vi "Teleop.vi"(10 "Match Info":T4={"Autonomous Elapsed Seconds"=0.0, "TeleOp Elapsed Seconds"=0.0, "Disabled Elapsed Seconds"=0.0, "Visited Autonomous"=FALSE, "Visited TeleOp"=FALSE, "Visited Disabled"=FALSE, "Autonomous Settings"={"Autonomous Style"=enum."Independent", "VI Refnum"=refnum}}, 11 "Call Context":T5) -> ()   [LabVIEW 2020]
doc: "This VI is called for each TeleOp packet received from the DS where the robot is not disabled. It is often used to read from the joysticks and update I/O or to update setpoints for timed control loops. It should complete and return within 20 milliseconds or it may miss DS packets."
uses:
  <vilib>/Rock Robotics/WPI/DriverStation/WPI_DriverStationDerivedRobotMode.ctl
  <vilib>/Rock Robotics/WPI/DriverStation/WPI_DriverStationMatch Info.ctl
  <vilib>/Rock Robotics/WPI/ThirdParty/REV Robotics/REVLib/Typedef/Color Sensor V3 Resolution.ctl
  <vilib>/Rock Robotics/WPI/ThirdParty/REV Robotics/REVLib/Typedef/Color Sensor V3 MeasurementRate.ctl
  <vilib>/Rock Robotics/WPI/ThirdParty/REV Robotics/REVLib/Typedef/Color Sensor V3 GainFactor.ctl
  <vilib>/Rock Robotics/WPI/ThirdParty/Phoenix-LabVIEW/Motor Controller/Controls/CTRE_Phoenix_MotorControl_ControlMode.ctl
  <vilib>/Rock Robotics/Network Tables/NT Read Boolean.vi
  <vilib>/Rock Robotics/Network Tables/NT Read Number.vi
  <vilib>/Rock Robotics/WPI/Utilities/WPI_GetSetVariantRefNum.vi
  GitHub/2022-Rapid-React-Code/TitanLib/Lib/TitanLib.lvlib
  <vilib>/Rock Robotics/WPI/ThirdParty/Phoenix-LabVIEW/CANCoder/Get/CTRE_Phoenix_CANcoder_GetSensorData.vi
panel:
  in  "Azimuth Limit":dbl(slide) scale=0.0..1.0
  in  "Drive Limit":dbl(slide) scale=0.0..1.0
  out "IR Detected":bool
  in  "Set":bool
  in  "GainFactor":T1
  in  "ColorSensorMeasurementRate":T2
  in  "ColorSensorResolution":T3
  in  "Red Calibration":cluster{"R":dbl, "G":dbl, "B":dbl}
  in  "Blue Calibration":cluster{"R":dbl, "G":dbl, "B":dbl}
  in  "Yellow Calibration":cluster{"R":dbl, "G":dbl, "B":dbl}
  in  "Green Calibration":cluster{"R":dbl, "G":dbl, "B":dbl}
  out "Proximity Chart":u16(graph)
  out "Confidence":dbl
  out "Matched Color Name":string
  out "error out":errorcluster
  out "Color":u32(colorbox)
  out "Measured Color":cluster{"R":dbl, "G":dbl, "B":dbl}
  out "Sample Slider 0":dbl(slide) scale=0.0..5.0
  out "Sample Boolean 1":bool
  out "Sample Boolean 0":bool
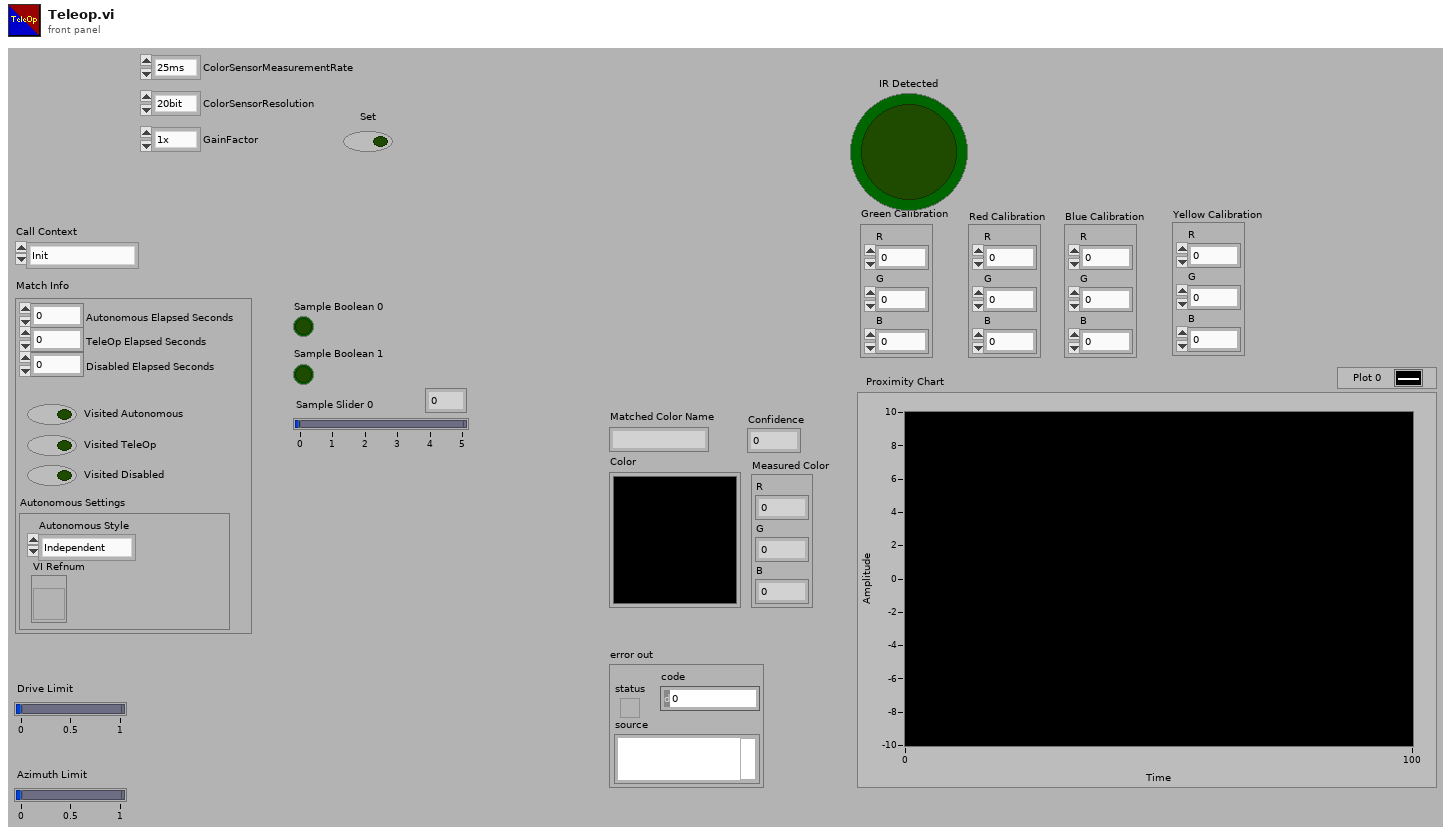
[diagram p1: front panel]
types:
  T1 = typedef "Color Sensor V3 GainFactor.ctl" = enum16{"1x", "3x", "6x", "9x", "18x"}
  T2 = typedef "Color Sensor V3 MeasurementRate.ctl" = enum16{"25ms", "50ms", "100ms", "200ms", "500ms", "1000ms", "2000ms"}
  T3 = typedef "Color Sensor V3 Resolution.ctl" = enum16{"20bit", "19bit", "18bit", "17bit", "16bit", "13bit"}
  T4 = typedef "WPI_DriverStationMatch Info.ctl" = cluster{"Autonomous Elapsed Seconds":dbl, "TeleOp Elapsed Seconds":dbl, "Disabled Elapsed Seconds":dbl, "Visited Autonomous":bool, "Visited TeleOp":bool, "Visited Disabled":bool, "Autonomous Settings":cluster{"Autonomous Style":enum16{"Iterative", "Independent"}, "VI Refnum":refnum<vi>}}
  T5 = typedef "WPI_DriverStationDerivedRobotMode.ctl" = enum16{"Init", "Execute", "Stop"}
  T6 = typedef "CTRE_Phoenix_MotorControl_ControlMode.ctl" = u16
  T7 = typedef "Color Sensor V3 DevRef.ctl" = cluster{"I2CDevRef":T8}
  T8 = typedef "WPI_I2CDevRef.ctl" = cluster{"DevStatus":errorcluster, "Device Address":u8, "Handle":i32, "I2C Bus":T9}
  T9 = typedef "i2c_bus.ctl" = enum16{"I2C On-Board", "I2C MXP", "Invalid"}
  T10 = typedef "WPI_DigitalInputDevRef.ctl" = cluster{"DevStatus":errorcluster, "DIO Channel":T11}
  T11 = typedef "FPGA_DIOChannel.ctl" = enum8{"DIO 0", "DIO 1", "DIO 2", "DIO 3", "DIO 4", "DIO 5", "DIO 6", "DIO 7", "DIO 8", "DIO 9", "DIO MXP 0", "DIO MXP 1", "DIO MXP 2", "DIO MXP 3", "DIO MXP 4", "DIO MXP 5", "DIO MXP 6", "DIO MXP 7", "DIO MXP 8", "DIO MXP 9", "DIO MXP 10", "DIO MXP 11", "DIO MXP 12", "DIO MXP 13", "DIO MXP 14", "DIO MXP 15", "SPI Port CS1", "SPI Port CS2", "SPI Port CS3", "SPI Port MISO", "SPI Port MOSI", "Invalid"}
  T12 = typedef "WPI_JoystickDevRef.ctl" = cluster{"Device":T13}
  T13 = typedef "WPI_JoystickDeviceEnum.ctl" = enum16{"USB 0", "USB 1", "USB 2", "USB 3", "USB 4", "USB 5"}
  T14 = typedef "CTRE_Phoenix_CANcoder_DeviceRef.ctl" = cluster{"DeviceStatus":errorcluster, "Device Number":u8, "Handle":u64, "UsageFrame":u32, "Library Path":path}
  T15 = typedef "WPI_MotorControlDeviceRef.ctl" = cluster{"DeviceStatus":errorcluster, "Type":T16, "PWM":cluster{"PWM Channel":T17, "DeadBand":T18}, "CAN":cluster{"Device Number":u8, "SetOutput VI Ref":variant, "GetOutput VI Ref":variant, "Enable VI Ref":variant, "Disable VI Ref":variant, "Data":variant}, "Invert":bool, "DIO PWM":cluster{"PWM \"Enable\" Channel":T17, "DIOChannel":T11, "PWM Rate":dbl}}
  T16 = typedef "WPI_MotorControlType.ctl" = enum16{"PWM", "CAN", "DIO PWM"}
  T17 = typedef "FPGA_DIOPWMChannel.ctl" = enum8{"PWM 0", "PWM 1", "PWM 2", "PWM 3", "PWM 4", "PWM 5", "PWM 6", "PWM 7", "PWM 8", "PWM 9", "PWM MXP 0", "PWM MXP 1", "PWM MXP 2", "PWM MXP 3", "PWM MXP 4", "PWM MXP 5", "PWM MXP 6", "PWM MXP 7", "PWM MXP 8", "PWM MXP 9", "Invalid"}
  T18 = typedef "WPI_PWMDeadband.ctl" = cluster{"Name":string, "maxPositivePwm":i32, "minPositivePwm":i32, "centerPwm":i32, "maxNegativePwm":i32, "minNegativePwm":i32, "angularRange":u16}
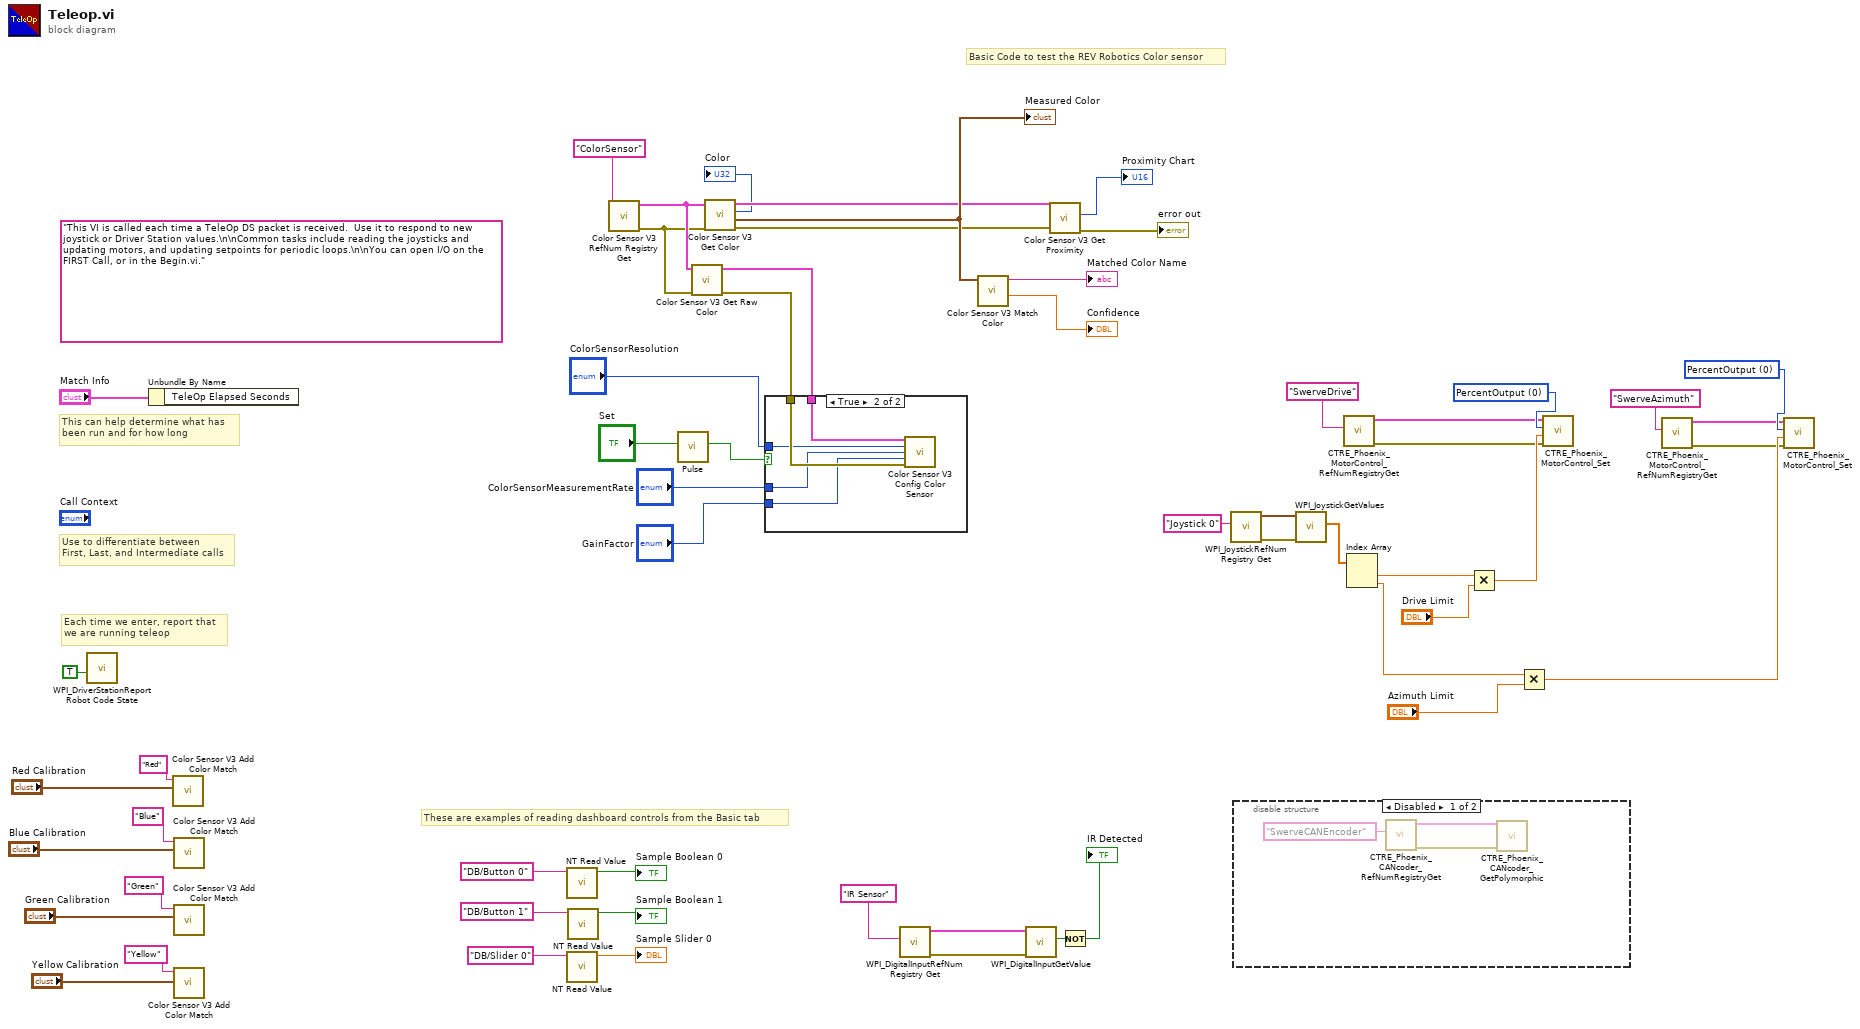
[diagram p0: block diagram]
diagram:
  w18 = T6 0 items=["PercentOutput"=0, "Position"=1, "Velocity"=2, "Current"=3, "Follower"=5, "MotionProfile"=6, "MotionMagic"=7, "MotionProfileArc"=10, "Disabled"=15] ("Control Mode")
  w17 = T6 0 items=["PercentOutput"=0, "Position"=1, "Velocity"=2, "Current"=3, "Follower"=5, "MotionProfile"=6, "MotionMagic"=7, "MotionProfileArc"=10, "Disabled"=15] ("Control Mode")
  (unwired) "This VI is called each time a TeleOp DS packet is received.  Use it to respond to new joystick or Driver Station values.\n\nCommon tasks include reading the joysticks and updating motors, and updating setpoints for periodic loops.\n\nYou can open I/O on the FIRST Call, or in the Begin.vi."
  # "Basic Code to test the REV Robotics Color sensor"
  # "These are examples of reading dashboard controls from the Basic tab"
  # "Each time we enter, report that\nwe are running teleop"
  # "Use to differentiate between\nFirst, Last, and Intermediate calls"
  # "This can help determine what has\nbeen run and for how long"
  n1 = call <vilib>:"WPI_DriverStationReport Robot Code State.vi"("TeleOp"=TRUE ("Autonomous")) -> ()  [unwired: 10 in, 1 out]
  n2 = Unbundle By Name("Match Info") -> ()  [unwired: 1 out]
  n3 = call <vilib>:"Color Sensor V3 Add Color Match.vi"("Color"="Red Calibration", "Name"="Red") -> ()  [unwired: 10 in]
  n4 = call <vilib>:"Color Sensor V3 Add Color Match.vi"("Color"="Blue Calibration", "Name"="Blue") -> ()  [unwired: 10 in]
  n5 = call <vilib>:"Color Sensor V3 Add Color Match.vi"("Color"="Green Calibration", "Name"="Green") -> ()  [unwired: 10 in]
  n6 = call <vilib>:"Color Sensor V3 Add Color Match.vi"("Color"="Yellow Calibration", "Name"="Yellow") -> ()  [unwired: 10 in]
  n7 = call-poly <vilib>:"NT Read Value.vi"("Name"="DB/Button 0" ("refnum name")) -> ("Boolean"=→"Sample Boolean 0":bool)  [unwired: 9 in, 1 out]
  n8 = call-poly <vilib>:"NT Read Value.vi"("Name"="DB/Slider 0" ("refnum name")) -> ("Numeric"=→"Sample Slider 0":dbl)  [unwired: 9 in, 1 out]
  n9 = call-poly <vilib>:"NT Read Value.vi"("Name"="DB/Button 1" ("refnum name")) -> ("Boolean"=→"Sample Boolean 1":bool)  [unwired: 9 in, 1 out]
  n10 = call <vilib>:"Color Sensor V3 RefNum Registry Get.vi"("refnum name"="ColorSensor") -> ("error out"=w31:errorcluster, "ColorSensorDevRef"=w32:T7)  [unwired: 9 in]
  n11 = call "Pulse.vi"("Input"="Set") -> ("Output"=w24:bool)  [unwired: 10 in]
  n12 = call <vilib>:"Color Sensor V3 Get Raw Color.vi"("error in (no error)"=w31, "ColorSensorDevRef"=w32) -> ("error out"=w30:errorcluster, "ColorSensorDevRef out"=w29:T7)  [unwired: 7 in, 1 out]
  n13 = call <vilib>:"Color Sensor V3 Get Color.vi"("error in (no error)"=w31, "ColorSensorDevRef"=w32) -> ("error out"=w38:errorcluster, "Normalized Color"=w40:cluster{"R":dbl, "G":dbl, "B":dbl}, "Color"=→"Color":u32, "ColorSensorDevRef out"=w39:T7)  [unwired: 6 in]
  "Measured Color" <- w40
  n14 = case shown="True" w24 {
    tunnel: w30 -> [_ w62]
    tunnel: w29 -> [_ w61]
    tunnel: "ColorSensorResolution" -> [_ w60]
    tunnel: "ColorSensorMeasurementRate" -> [_ w59]
    tunnel: "GainFactor" -> [_ w58]
    frame False {
    }
    frame True {
      n15 = call <vilib>:"Color Sensor V3 Config Color Sensor.vi"("ColorSensorDevRef"=w61, "ColorSensorResolution"=w60, "ColorSensorMeasurementRate"=w59, "GainFactor"=w58, "error in (no error)"=w62) -> ()  [unwired: 9 in, 2 out]
    }
  }
  n16 = call <vilib>:"WPI_DigitalInputRefNum Registry Get.vi"("refnum name"="IR Sensor") -> ("error out"=w23:errorcluster, "DigitalInputDevRef"=w22:T10)  [unwired: 9 in]
  n17 = call <vilib>:"Color Sensor V3 Match Color.vi"("Measured Color"=w40) -> ("Confidence"=→"Confidence":dbl, "Matched Color Name"=→"Matched Color Name":string)  [unwired: 8 in, 1 out]
  n18 = call <vilib>:"WPI_DigitalInputGetValue.vi"("error in (no error)"=w23, "DigitalInputDevRef"=w22) -> ("Value"=w21:bool)  [unwired: 7 in, 2 out]
  n19 = call <vilib>:"Color Sensor V3 Get Proximity.vi"("error in (no error)"=w38, "ColorSensorDevRef"=w39) -> ("error out"=→"error out":errorcluster, "Proximity"=→"Proximity Chart":u16)  [unwired: 7 in, 1 out]
  n20 = Not(x=w21) -> (.not. x?=→"IR Detected":bool)
  n21 = call <vilib>:"WPI_JoystickRefNum Registry Get.vi"("refnum name"="Joystick 0") -> ("error out"=w2:errorcluster, "JoystickDevRef"=w3:T12)  [unwired: 9 in]
  n22 = disable-structure shown="Disabled" {
    frame Disabled {
      n23 = call <vilib>:"CTRE_Phoenix_CANcoder_RefNumRegistryGet.vi"("refnum name"="SwerveCANEncoder") -> ("error out"=w63:errorcluster, "CTRE_CANcoder_DeviceRef"=w64:T14)  [unwired: 9 in]
      n24 = call-poly <vilib>:"CTRE_Phoenix_CANcoder_GetPolymorphic.vi"("CTRE_CANcoder_DeviceRef"=w64, "error in"=w63) -> ()  [unwired: 9 in, 5 out]
    }
    frame Enabled {
    }
  }
  n25 = call <vilib>:"WPI_JoystickGetValues.vi"("error in (no error)"=w2, "JoystickDevRef"=w3) -> ("Axes"=w4:dbl[])  [unwired: 5 in, 4 out]
  n26 = call <vilib>:"CTRE_Phoenix_MotorControl_RefNumRegistryGet.vi"("refnum name"="SwerveDrive") -> ("error out"=w5:errorcluster, "PhoenixMotorControlDevRef"=w6:T15)  [unwired: 9 in]
  n27 = Index Array(array=w4) -> (element #1=w8:dbl, element #2=w14:dbl)  [unwired: 2 in]
  n28 = Multiply(x=w8, y="Drive Limit") -> (x*y=w10:dbl)
  n29 = Multiply(x=w14, y="Azimuth Limit") -> (x*y=w15:dbl)
  n30 = call <vilib>:"CTRE_Phoenix_MotorControl_Set.vi"("error in (no error)"=w5, "Output"=w10, "Control Mode"=w17, "PhoenixMotorControlDevRef"=w6) -> ()  [unwired: 6 in, 2 out]
  n31 = call <vilib>:"CTRE_Phoenix_MotorControl_RefNumRegistryGet.vi"("refnum name"="SwerveAzimuth") -> ("error out"=w11:errorcluster, "PhoenixMotorControlDevRef"=w12:T15)  [unwired: 9 in]
  n32 = call <vilib>:"CTRE_Phoenix_MotorControl_Set.vi"("error in (no error)"=w11, "Output"=w15, "Control Mode"=w18, "PhoenixMotorControlDevRef"=w12) -> ()  [unwired: 6 in, 2 out]
